vi "Tach RPM_FPGA.vi"() -> ()   [LabVIEW 2010]
uses:
  <vilib>/eio/EIONode/EIONode.xnode
  <vilib>/rvi/eio/nirviEIOImplementation/nirviEIOImplementation.xnode
  <vilib>/rvi/eio/common/nirviEmuClasses.ctl
  <vilib>/rvi/eio/common/nirviEmuTemplateMethod_noerrors.vi
panel:
  out "Analog In (Tach)":fxp<+/-,24,4> format="%.22g"
  in  "Threshold":fxp<+/-,16,16>
  in  "Hysteresis":fxp<+,1,0>=0.5 format="%.1g"
  out "Tach State":enum16{"Check Hysteresis", "Check Threshold"}(ring)
  out "Tach Period (uSec/pulse)":u32
  in  "Slope":enum16{"falling", "rising"}(ring)=enum."rising"
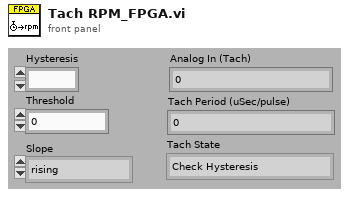
[diagram p1: front panel]
types:
  T1 = typedef "nirviEmuClasses.ctl" = enum16{"IO Read", "IO Write", "Method", "Property Read", "Property Write"}
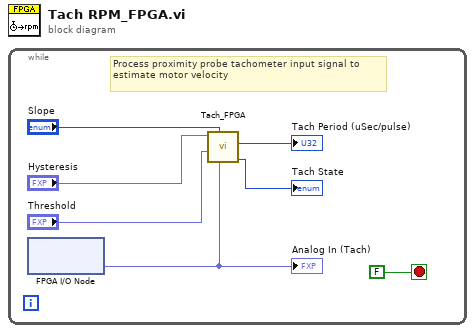
[diagram p0: block diagram]
diagram:
  n1 = while {
    stop <- FALSE stop-if-true
    # "Process proximity probe tachometer input signal to estimate motor velocity"
    n2 = xnode "FPGA I/O Node"() -> ("Tach0"=w5:fxp<+/-,24,4>)  [unwired: 1 in, 1 out]
    "Analog In (Tach)" <- w5
    n3 = call "Tach_FPGA.vi"("Analog In (Tach)"=w5, "Slope"="Slope", "Threshold"="Threshold", "Hysteresis"="Hysteresis") -> ("Tach State"=→"Tach State":enum16{"Check Hysteresis", "Check Threshold"}, "Tach Period (uSec/pulse)"=→"Tach Period (uSec/pulse)":u32)  [unwired: 6 in]
  }
